vi "Convert from JSON Comp Format.vi"(11 "JSON format":T6) -> (3 "digital audio protocol settings":T1={"number of channels"=0, "data justification"=enum."Left Justified", "endianness"=enum."LSB First", "channel length"=0, "bit depth"=0, "frame clock rate"=0.0, "bit clock edge sync"=enum."Falling", "master clock rate"=0.0, "Logic Level"=enum."1.2 V", "frame sync edge for channel 0"=enum."Rising", "Channel 0 Offset"=0})   [LabVIEW 2021, in "digital audio protocol controls.lvlib"]
uses:
  digital audio protocol controls.lvlib
  digital audio protocol settings_json.ctl
  digital audio protocol settings.ctl
  <vilib>/PDM Acquisition Toolkit/shared/controls/PCM Data Justification.ctl
  <vilib>/PDM Acquisition Toolkit/shared/controls/PCM Bit Endianness.ctl
  <vilib>/PDM Acquisition Toolkit/shared/controls/Digital Edge.ctl
  <vilib>/PDM Acquisition Toolkit/host/Classes/Session/Controls/Logic Levels.ctl
  <vilib>/PDM Acquisition Toolkit/shared/PDM Shared.lvlib
  <vilib>/PDM Acquisition Toolkit/host/Classes/Session/DecoderSession.lvclass
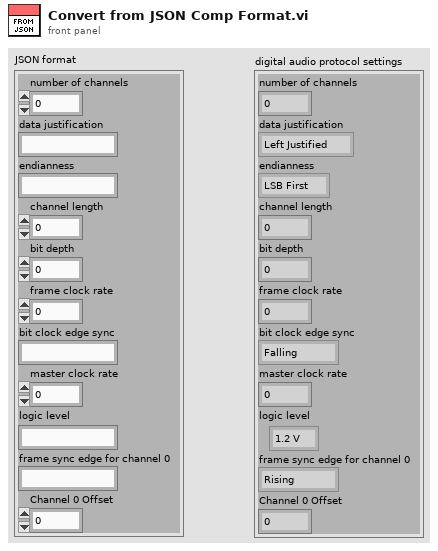
[diagram p1: front panel]
types:
  T1 = typedef "digital audio protocol controls.lvlib/digital audio protocol settings.ctl" = cluster{"number of channels":u32, "data justification":T2, "endianness":T3, "channel length":u32, "bit depth":u32, "frame clock rate":dbl, "bit clock edge sync":T4, "master clock rate":dbl, "Logic Level":T5, "frame sync edge for channel 0":T4, "Channel 0 Offset":u32}
  T2 = typedef "PDM Shared.lvlib/PCM Data Justification.ctl" = enum16{"Left Justified", "Right Justified"}
  T3 = typedef "PDM Shared.lvlib/PCM Bit Endianness.ctl" = enum16{"MSB First", "LSB First"}
  T4 = typedef "PDM Shared.lvlib/Digital Edge.ctl" = enum8{"Rising", "Falling"}
  T5 = typedef "PDM Acquisition Class Library.lvlib/DecoderSession.lvclass/Logic Levels.ctl" = enum16{"3.3 V", "1.8 V", "1.2 V"}
  T6 = typedef "digital audio protocol controls.lvlib/digital audio protocol settings_json.ctl" = cluster{"number of channels":u32, "data justification":string, "endianness":string, "channel length":u32, "bit depth":u32, "frame clock rate":dbl, "bit clock edge sync":string, "master clock rate":dbl, "logic level":string, "frame sync edge for channel 0":string, "Channel 0 Offset":u32}
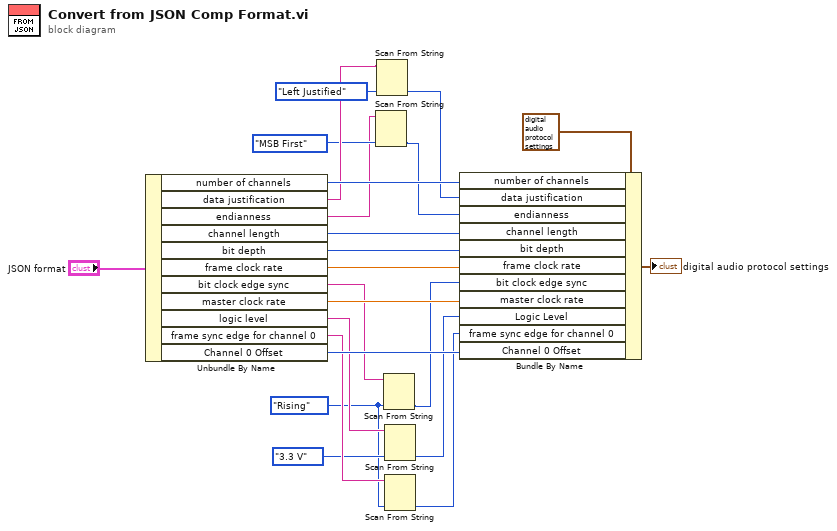
[diagram p0: block diagram]
diagram:
  w4 = Digital_Edge."Rising" ("bit clock edge sync")
  n1 = Unbundle By Name("JSON format") -> ("number of channels"=w23:u32, "data justification"=w14:string, "endianness"=w10:string, "channel length"=w22:u32, "bit depth"=w21:u32, "frame clock rate"=w20:dbl, "bit clock edge sync"=w8:string, "master clock rate"=w19:dbl, "logic level"=w7:string, "frame sync edge for channel 0"=w6:string, "Channel 0 Offset"=w18:u32)
  n2 = Scan From String(input string=w10, default 1=PCM_Bit_Endianness."MSB First" ("endianness")) -> (output 1=w9:T3)  [unwired: 3 in, 3 out]
  n3 = Scan From String(input string=w14, default 1=PCM_Data_Justification."Left Justified" ("data justification")) -> (output 1=w12:T2)  [unwired: 3 in, 3 out]
  n4 = Scan From String(input string=w8, default 1=w4) -> (output 1=w3:T4)  [unwired: 3 in, 3 out]
  n5 = Scan From String(input string=w7, default 1=Logic_Levels."3.3 V" ("Logic Level")) -> (output 1=w2:T5)  [unwired: 3 in, 3 out]
  n6 = Scan From String(input string=w6, default 1=w4) -> (output 1=w1:T4)  [unwired: 3 in, 3 out]
  n7 = Bundle By Name(cluster=T1 {"number of channels"=0, "data justification"=enum."Left Justified", "endianness"=enum."LSB First", "channel length"=0, "bit depth"=0, "frame clock rate"=0.0, "bit clock edge sync"=enum."Falling", "master clock rate"=0.0, "Logic Level"=enum."1.2 V", "frame sync edge for channel 0"=enum."Rising", "Channel 0 Offset"=0} ("digital audio protocol settings"), "number of channels"=w23, "data justification"=w12, "endianness"=w9, "channel length"=w22, "bit depth"=w21, "frame clock rate"=w20, "bit clock edge sync"=w3, "master clock rate"=w19, "Logic Level"=w2, "frame sync edge for channel 0"=w1, "Channel 0 Offset"=w18) -> (→"digital audio protocol settings":T1)
